vi "IMAQController.CalculateGrid.vi"(1 "Central":i32, 2 "PixelDistanceBetweenGridLines":dbl, 3 "AxesMin":i32, 4 "AxesMax":i32) -> (16 "sorted array":i32[](array[numeric]), 18 "Error":bool)   [LabVIEW 2014, in "IMAQController.lvlib"]
uses:
  IMAQController.lvlib
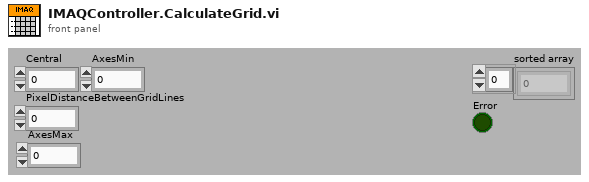
[diagram p1: front panel]
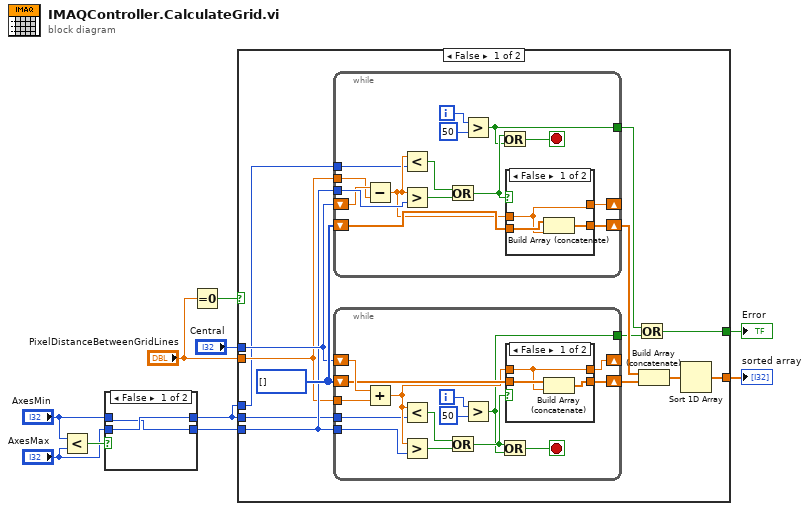
[diagram p0: block diagram]
diagram:
  n1 = Less?(x="AxesMin", y="AxesMax") -> (x < y?=w6:bool)
  n2 = case shown="False" w6 {
    tunnel: [w11 w14] -> w5
    tunnel: "AxesMax" -> [w12 w14]
    tunnel: [w12 w13] -> w3
    tunnel: "AxesMin" -> [w11 w13]
    frame False {
    }
    frame True {
    }
  }
  n3 = Equal To 0?(x="PixelDistanceBetweenGridLines") -> (x = 0?=w7:bool)
  n4 = case shown="False" w7 {
    tunnel: [w23 _] -> w10
    tunnel: "Central" -> [w22 _]
    tunnel: w5 -> [w21 _]
    tunnel: "PixelDistanceBetweenGridLines" -> [w20 _]
    tunnel: w3 -> [w19 _]
    tunnel: w3 -> [w18 _]
    tunnel: [w15 _] -> w1
    frame False {
      w27 = i32[] []
      n5 = while {
        tunnel: w21 -> [w60]
        shift-right: [w55] -> w25
        shift-left: w27 -> [w57]
        shift-right: [w56] -> _
        shift-left: w22 -> [w59]
        tunnel: w20 -> [w58]
        tunnel: w19 -> [w53]
        tunnel: [w48] -> w16
        i -> [w50]
        stop <- w51 stop-if-true
        n6 = Subtract(x=w59, y=w58) -> (x-y=w54:dbl)
        n7 = Less?(x=w54, y=w53) -> (x < y?=w62:bool)
        n8 = Greater?(x=w54, y=w60) -> (0:w61:bool)
        n9 = Or(x=w62, y=w61) -> (x .or. y?=w52:bool)
        n10 = Greater?(x=w50, y=50) -> (0:w48:bool)
        n11 = Or(x=w52, y=w48) -> (x .or. y?=w51:bool)
        n12 = case shown="False" w52 {
          tunnel: w57 -> [w65 w66]
          tunnel: w54 -> [w63 w67]
          tunnel: [w63 w67] -> w56
          tunnel: [w64 w66] -> w55
          frame False {
            n13 = Build Array (concatenate)(w65, w63) -> (w64:dbl[])
          }
          frame True {
          }
        }
      }
      n14 = while {
        tunnel: w21 -> [w40]
        shift-right: [w35] -> w26
        shift-left: w27 -> [w37]
        shift-right: [w36] -> _
        shift-left: w22 -> [w39]
        tunnel: w20 -> [w38]
        tunnel: w18 -> [w33]
        tunnel: [w28] -> w17
        i -> [w29]
        stop <- w30 stop-if-true
        n15 = Add(x=w39, y=w38) -> (x+y=w34:dbl)
        n16 = Less?(x=w34, y=w33) -> (x < y?=w42:bool)
        n17 = Greater?(x=w34, y=w40) -> (0:w41:bool)
        n18 = Or(x=w42, y=w41) -> (x .or. y?=w31:bool)
        n19 = Greater?(x=w29, y=50) -> (0:w28:bool)
        n20 = Or(x=w31, y=w28) -> (x .or. y?=w30:bool)
        n21 = case shown="False" w31 {
          tunnel: w37 -> [w45 w46]
          tunnel: w34 -> [w43 w47]
          tunnel: [w43 w47] -> w36
          tunnel: [w44 w46] -> w35
          frame False {
            n22 = Build Array (concatenate)(w45, w43) -> (w44:dbl[])
          }
          frame True {
          }
        }
      }
      n23 = Or(x=w16, y=w17) -> (x .or. y?=w15:bool)
      n24 = Build Array (concatenate)(w25, w26) -> (w24:dbl[])
      n25 = Sort 1D Array(array=w24) -> (sorted array=w23:dbl[])
    }
    frame True {
    }
  }
  "sorted array" <- w10
  "Error" <- w1
